vi "close livedata displays.vi"(11 "messageHandler in":T1 {"params"."controlChannels"."ballControl" items=["Module6/output0", "Module6/output1", "Module6/output2", "Module6/output3", "Not-Used"]; "params"."controlChannels"."butterflyControl" items=["Module6/output0", "Module6/output1", "Module6/output2", "Module6/output3", "Not-Used"]; "params"."controlChannels"."speedControl" items=["Module6/output0", "Module6/output1", "Module6/output2", "Module6/output3", "Not-Used"]}) -> (3 "messageHandler out":T1 {"params"."controlChannels"."ballControl" items=["Module6/output0", "Module6/output1", "Module6/output2", "Module6/output3", "Not-Used"]; "params"."controlChannels"."butterflyControl" items=["Module6/output0", "Module6/output1", "Module6/output2", "Module6/output3", "Not-Used"]; "params"."controlChannels"."speedControl" items=["Module6/output0", "Module6/output1", "Module6/output2", "Module6/output3", "Not-Used"]})   [LabVIEW 2018]
uses:
  type defs/message handler data.ctl
  customVI/liveData/state.ctl
types:
  T1 = typedef "message handler data.ctl" = cluster{"params":cluster{"configFileID":u32, "configFilePath":path, "channelConfigFilePath":path, "incidentLogfile":path, "controlChannels":cluster{"ballControl":u16, "butterflyControl":u16, "speedControl":u16}, "pulsatorVIPath":path, "customVIPath":path, "HowdenAir":cluster{"vent Howden":bool, "Howden%":dbl}}, "vars":cluster{"commsStatus":bool[], "controlIndex":cluster{"ballControl":u16, "butterflyControl":u16, "speedControl":u16}, "customVIRef":refnum<vi>, "Interlocks":cluster{"gearboxOil":bool, "bearingOil":bool, "gearboxAir":bool}, "motorRunning":bool, "liveDataQ":refnum<queue>[]}}
  T2 = typedef "state.ctl" = enum16{"readData", "init", "channel", "mode", "quit"}
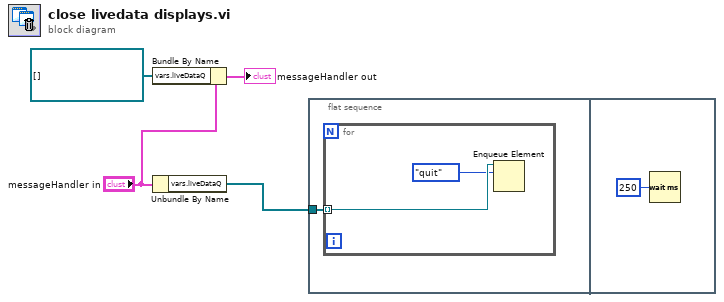
[diagram p0: block diagram]
diagram:
  w1 = refnum<queue>[] [] items=["readData", "init", "channel", "mode", "quit"] ("vars.liveDataQ")
  n1 = Bundle By Name(cluster="messageHandler in", "vars.liveDataQ"=w1) -> (→"messageHandler out":T1)
  n2 = Unbundle By Name("messageHandler in") -> ("vars.liveDataQ"=w4:refnum<queue>[])
  n3 = flat-sequence {
    tunnel: w4 -> [w5]
    frame #0 {
      n4 = for {
        tunnel: w5 -> [w7] mode=indexing
        n5 = Enqueue Element(queue=w7, element=state."quit") -> ()  [unwired: 2 in, 3 out]
      }
    }
    frame #1 {
      n6 = Wait (ms)(milliseconds to wait=u32 250) -> ()  [unwired: 1 out]
    }
  }
